vi "appendNewTransactions.vi"(8 "error in (no error)":errorcluster, 10 "TransactionList.lvclass":refnum<class "TransactionList.lvclass">, 11 "Database in":refnum<class "Account History.lvclass">) -> (0 "error out":errorcluster, 1 "Num records":i32, 3 "Database out":refnum<class "Account History.lvclass">)   [LabVIEW 2020, in "Account History.lvclass"]
uses:
  Account History.lvclass
  Statement/TransactionList.lvclass
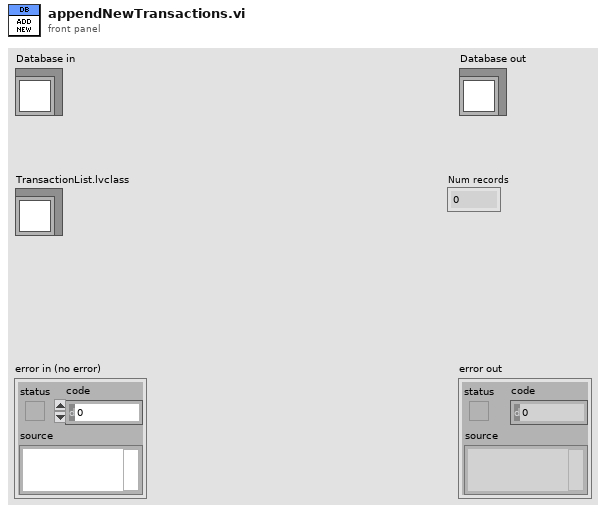
[diagram p1: front panel]
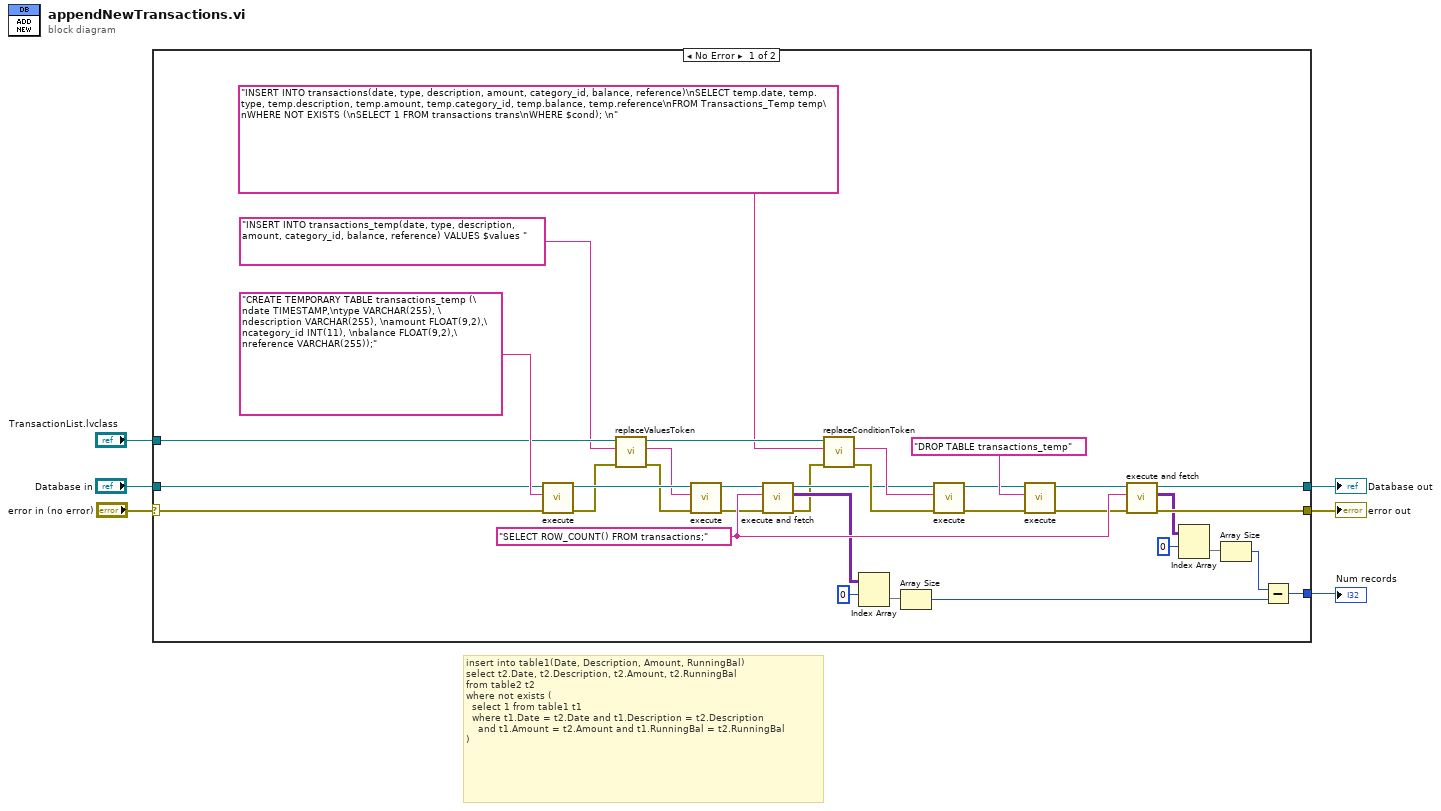
[diagram p0: block diagram]
diagram:
  # "insert into table1(Date, Description, Amount, RunningBal)\nselect t2.Date, t2.Description, t2.Amount, t2.RunningBal\nfrom table2 t2\nwhere not exists (\n  select 1 from table1 t1\n  where t1.Date = t2.Date and t1.Description = t2.Description\n    and t1.Amount = t2.Amount and t1.RunningBal = t2.RunningBal\n)"
  n1 = case shown="No Error" "error in (no error)" {
    selector: "error in (no error)" -> [w10 w41]
    tunnel: "Database in" -> [w7 w42]
    tunnel: [w37 w42] -> w5
    tunnel: [w36 w41] -> w4
    tunnel: "TransactionList.lvclass" -> [w29 _]
    tunnel: [w40 _] -> w2
    frame No Error {
      w35 = "SELECT ROW_COUNT() FROM transactions;" ("SQL query")
      n2 = call "execute.vi"("error in (no error)"=w10, "SQL query"="CREATE TEMPORARY TABLE transactions_temp (\ndate TIMESTAMP,\ntype VARCHAR(255), \ndescription VARCHAR(255), \namount FLOAT(9,2),\ncategory_id INT(11), \nbalance FLOAT(9,2),\nreference VARCHAR(255));", "Database in"=w7) -> ("error out"=w27:errorcluster, "Database out"=w38:refnum<class "Account History.lvclass">)  [unwired: 7 in]
      n3 = call "replaceValuesToken.vi"("error in (no error)"=w27, "Query"="INSERT INTO transactions_temp(date, type, description, amount, category_id, balance, reference) VALUES $values ", "TransactionList in"=w29) -> ("error out"=w26:errorcluster, "Query"=w28:string, "TransactionList out"=w24:refnum<class "TransactionList.lvclass">)  [unwired: 6 in]
      n4 = call "execute.vi"("error in (no error)"=w26, "SQL query"=w28, "Database in"=w38) -> ("error out"=w12:errorcluster, "Database out"=w11:refnum<class "Account History.lvclass">)  [unwired: 7 in]
      n5 = call "execute and fetch.vi"("error in (no error)"=w12, "SQL query"=w35, "Database in"=w11) -> ("error out"=w8:errorcluster, "recordset data"=w20:variant[][], "Database out"=w9:refnum<class "Account History.lvclass">)  [unwired: 6 in]
      n6 = call-dynamic "replaceConditionToken.vi"("error in (no error)"=w8, "Query In"="INSERT INTO transactions(date, type, description, amount, category_id, balance, reference)\nSELECT temp.date, temp.type, temp.description, temp.amount, temp.category_id, temp.balance, temp.reference\nFROM Transactions_Temp temp\nWHERE NOT EXISTS (\nSELECT 1 FROM transactions trans\nWHERE $cond); \n", "TransactionList in"=w24) -> ("error out"=w22:errorcluster, "Query Out"=w21:string)  [unwired: 6 in, 1 out]
      n7 = Index Array(array=w20, index (row)=0) -> (element=w19:variant[])  [unwired: 1 in]
      n8 = Array Size(array=w19) -> (size(s)=w17:i32)
      n9 = call "execute.vi"("error in (no error)"=w22, "SQL query"=w21, "Database in"=w9) -> ("error out"=w32:errorcluster, "Database out"=w33:refnum<class "Account History.lvclass">)  [unwired: 7 in]
      n10 = call "execute.vi"("error in (no error)"=w32, "SQL query"="DROP TABLE transactions_temp", "Database in"=w33) -> ("error out"=w30:errorcluster, "Database out"=w31:refnum<class "Account History.lvclass">)  [unwired: 7 in]
      n11 = call "execute and fetch.vi"("error in (no error)"=w30, "SQL query"=w35, "Database in"=w31) -> ("error out"=w36:errorcluster, "recordset data"=w14:variant[][], "Database out"=w37:refnum<class "Account History.lvclass">)  [unwired: 6 in]
      n12 = Index Array(array=w14, index (row)=0) -> (element=w16:variant[])  [unwired: 1 in]
      n13 = Array Size(array=w16) -> (size(s)=w13:i32)
      n14 = Subtract(x=w13, y=w17) -> (x-y=w40:i32)
    }
    frame Error {
    }
  }
  "error out" <- w4
  "Database out" <- w5
  "Num records" <- w2
